vi "Sensor HW Read.vi"(8 "Error":errorcluster, 9 "CloseLoop":bool, 11 "PhoenixMotorControlDevRef":T1) -> (0 "Error Out":errorcluster, 2 "Sensor Values Out":T6, 3 "DevRef Out":T1)   [LabVIEW 2023, in "Shooter FX_ACT.lvlib"]
uses:
  Shooter FX_ACT.lvlib
  <vilib>/Rock Robotics/WPI/MotorControl/WPI_MotorControlDeviceRef.ctl
  <vilib>/Rock Robotics/WPI/MotorControl/WPI_MotorControlType.ctl
  <vilib>/Rock Robotics/SystemInterfaces/DIO/FPGA_DIOPWMChannel.ctl
  <vilib>/Rock Robotics/WPI/PWM/WPI_PWMDeadband.ctl
  <vilib>/Rock Robotics/SystemInterfaces/DIO/FPGA_DIOChannel.ctl
  Shared Code/TypeDefs/Cluster_FX CloseLoop Values.ctl
  Shared Code/TypeDefs/Cluster_FX Sensor Values.ctl
  Shared Code/TypeDefs/Cluster_FX Current Values.ctl
  Shared Code/TypeDefs/Cluster_FX Voltage Values.ctl
  Cluster_HW Output Values.ctl
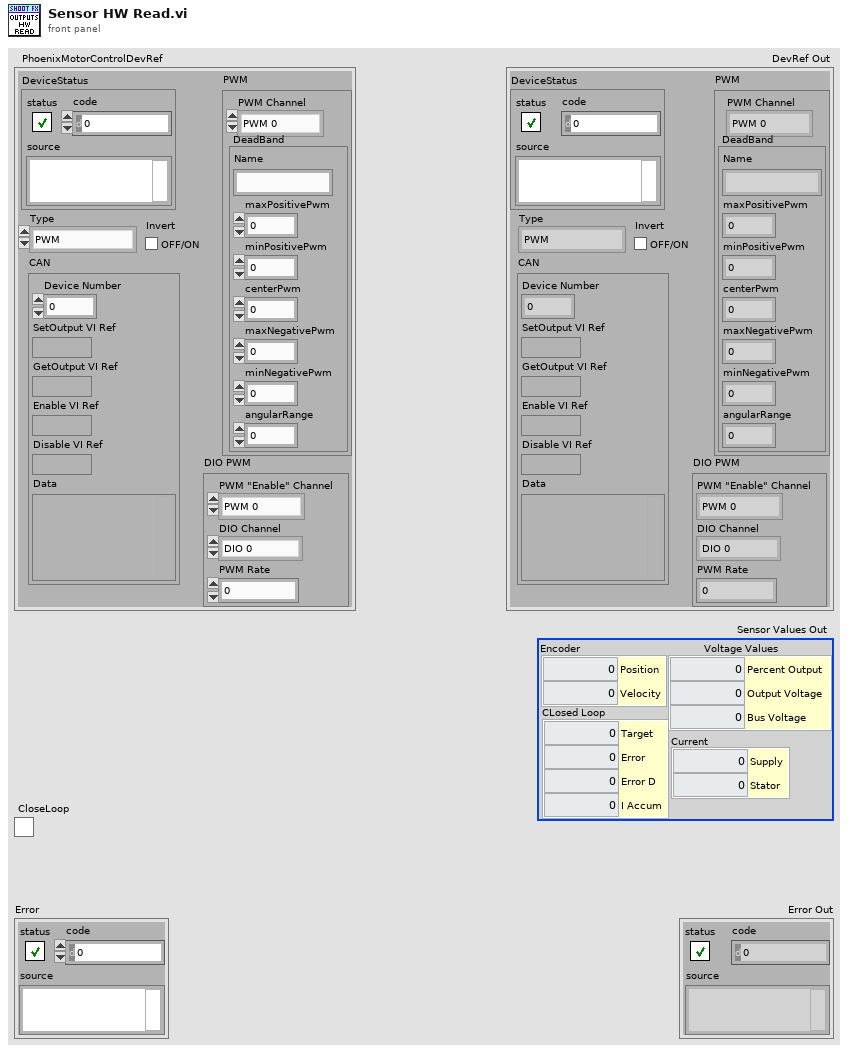
[diagram p1: front panel]
types:
  T1 = typedef "WPI_MotorControlDeviceRef.ctl" = cluster{"DeviceStatus":errorcluster, "Type":T2, "PWM":cluster{"PWM Channel":T3, "DeadBand":T4}, "CAN":cluster{"Device Number":u8, "SetOutput VI Ref":variant, "GetOutput VI Ref":variant, "Enable VI Ref":variant, "Disable VI Ref":variant, "Data":variant}, "Invert":bool, "DIO PWM":cluster{"PWM \"Enable\" Channel":T3, "DIOChannel":T5, "PWM Rate":dbl}}
  T2 = typedef "WPI_MotorControlType.ctl" = enum16{"PWM", "CAN", "DIO PWM"}
  T3 = typedef "FPGA_DIOPWMChannel.ctl" = enum8{"PWM 0", "PWM 1", "PWM 2", "PWM 3", "PWM 4", "PWM 5", "PWM 6", "PWM 7", "PWM 8", "PWM 9", "PWM MXP 0", "PWM MXP 1", "PWM MXP 2", "PWM MXP 3", "PWM MXP 4", "PWM MXP 5", "PWM MXP 6", "PWM MXP 7", "PWM MXP 8", "PWM MXP 9", "Invalid"}
  T4 = typedef "WPI_PWMDeadband.ctl" = cluster{"Name":string, "maxPositivePwm":i32, "minPositivePwm":i32, "centerPwm":i32, "maxNegativePwm":i32, "minNegativePwm":i32, "angularRange":u16}
  T5 = typedef "FPGA_DIOChannel.ctl" = enum8{"DIO 0", "DIO 1", "DIO 2", "DIO 3", "DIO 4", "DIO 5", "DIO 6", "DIO 7", "DIO 8", "DIO 9", "DIO MXP 0", "DIO MXP 1", "DIO MXP 2", "DIO MXP 3", "DIO MXP 4", "DIO MXP 5", "DIO MXP 6", "DIO MXP 7", "DIO MXP 8", "DIO MXP 9", "DIO MXP 10", "DIO MXP 11", "DIO MXP 12", "DIO MXP 13", "DIO MXP 14", "DIO MXP 15", "SPI Port CS1", "SPI Port CS2", "SPI Port CS3", "SPI Port MISO", "SPI Port MOSI", "Invalid"}
  T6 = typedef "Shooter FX_ACT.lvlib/Cluster_HW Output Values.ctl" = cluster{"Encoder":T7, "Current":T8, "CLosed Loop":T9, "Voltage Values":T10}
  T7 = typedef "Cluster_FX Sensor Values.ctl" = cluster{"Position":i32, "Velocity":i32}
  T8 = typedef "Cluster_FX Current Values.ctl" = cluster{"Supply":dbl, "Stator":dbl}
  T9 = typedef "Cluster_FX CloseLoop Values.ctl" = cluster{"Target":dbl, "Error":i32, "Error D":dbl, "I Accum":dbl}
  T10 = typedef "Cluster_FX Voltage Values.ctl" = cluster{"Percent Output":dbl, "Output Voltage":dbl, "Bus Voltage":dbl}
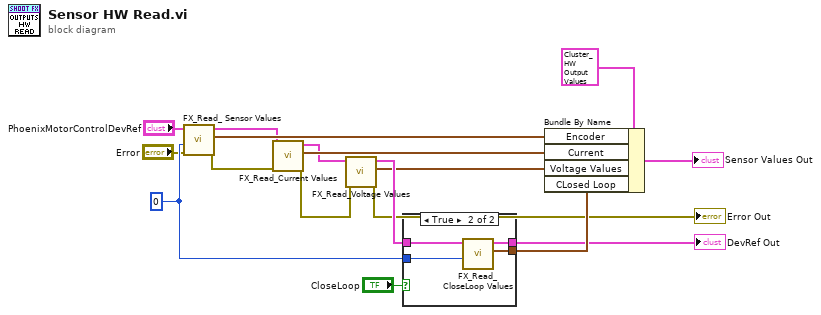
[diagram p0: block diagram]
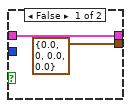
[diagram p2: hidden frame]
diagram:
  w10 = u32 0 ("PidLoopIdx")
  n1 = call "FX_Read_ Sensor Values.vi"("Error"="Error", "PidLoopIdx"=w10, "PhoenixMotorControlDevRef"="PhoenixMotorControlDevRef") -> ("Error Out"=w2:errorcluster, "Encoder Values Out"=w17:T7, "PhoenixMotorControlDevRef Out"=w1:T1)  [unwired: 6 in]
  n2 = call "FX_Read_Current Values.vi"("error in"=w2, "PhoenixMotorControlDevRef in"=w1) -> ("error out"=w12:errorcluster, "Current Values"=w16:T8, "PhoenixMotorControlDevRef out"=w14:T1)  [unwired: 7 in]
  n3 = call "FX_Read_Voltage Values.vi"("Error"=w12, "PhoenixMotorControlDevRef"=w14) -> ("Error Out"=→"Error Out":errorcluster, "Voltage Cluster Out"=w11:T10, "PhoenixMotorControlDevRef Out"=w13:T1)  [unwired: 7 in]
  n4 = case shown="True" "CloseLoop" {
    tunnel: w13 -> [w19 w23]
    tunnel: [w19 w22] -> w7
    tunnel: [T9 {"Target"=0.0, "Error"=0, "Error D"=0.0, "I Accum"=0.0} ("CLosed Loop Out") w21] -> w15
    tunnel: w10 -> [_ w20]
    frame False {
    }
    frame True {
      n5 = call "FX_Read_CloseLoop Values.vi"("Slot"=w20, "PhoenixMotorControlDevRef"=w23) -> ("CLosed Loop Out"=w21:T9, "PhoenixMotorControlDevRef Out"=w22:T1)  [unwired: 7 in, 1 out]
    }
  }
  "DevRef Out" <- w7
  n6 = Bundle By Name(cluster=T6 {"Encoder"={"Position"=0, "Velocity"=0}, "Current"={"Supply"=0.0, "Stator"=0.0}, "CLosed Loop"={"Target"=0.0, "Error"=0, "Error D"=0.0, "I Accum"=0.0}, "Voltage Values"={"Percent Output"=0.0, "Output Voltage"=0.0, "Bus Voltage"=0.0}} ("Sensor Values Out"), "Encoder"=w17, "Current"=w16, "Voltage Values"=w11, "CLosed Loop"=w15) -> (→"Sensor Values Out":T6)
